vi "Load Ini FIle.vi"(8 "error in (no error)":errorcluster, 10 "Variant":variant, 11 "configuration file path":path) -> (0 "error out":errorcluster, 3 "Array":string[](array[string]))   [LabVIEW 2019, in "Configuration.lvlib"]
doc: "This method decodes a ini file based on an example typedef."
uses:
  Configuration.lvlib
  <vilib>/Utility/config.llb/Read Key (U32).vi
  <vilib>/Utility/config.llb/Read Key (Boolean).vi
  <vilib>/Utility/config.llb/Read Key (String).vi
  <vilib>/Utility/config.llb/Read Key (Path).vi
  <vilib>/Utility/config.llb/Read Key (I32).vi
  <vilib>/Utility/config.llb/Read Key (Double).vi
  <vilib>/Utility/config.llb/NI_LVConfig.lvlib
  <vilib>/Utility/Data Type/NI_Data Type.lvlib
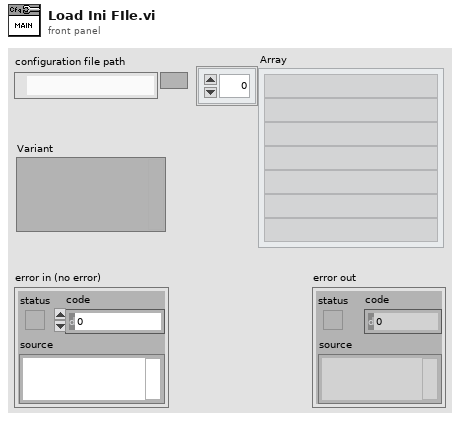
[diagram p1: front panel]
types:
  T1 = typedef "NI_LVConfig.lvlib/Config Data RefNum.ctl" = refnum<k1>
  T2 = typedef "NI_Data Type.lvlib/Data Type.ctl" = enum8{"Invalid Type", "Void", "I8", "I16", "I32", "I64", "U8", "U16", "U32", "U64", "Single Float", "Double Float", "Extended Float", "Single Complex", "Double Complex", "Extended Complex", "Enum U8", "Enum U16", "Enum U32", "Enum U64", "Single Float With Unit", "Double Float With Unit", "Extended Float With Unit", "Single Complex with Unit", "Double Complex with Unit", "Extended Complex with Unit", "Boolean", "String", "Path", "Picture", "Tag", "Array", "Cluster", "Variant", "LV Variant", "Waveform", "Timestamp", "Digital Waveform", "Digital Data", "ExpressData", "Refnum", "External Data", "VI", "Poly VI", "LabVIEW Class Instance", "Fixed Point", "Set Collection", "Map Collection"}
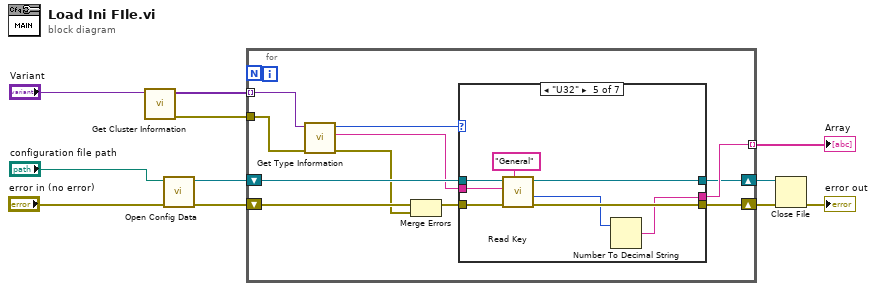
[diagram p0: block diagram]
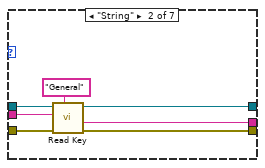
[diagram p3: hidden frame]
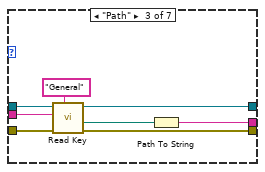
[diagram p4: hidden frame]
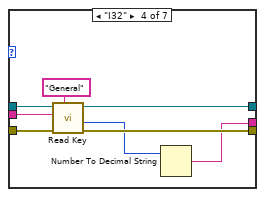
[diagram p5: hidden frame]
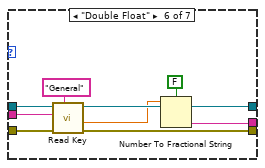
[diagram p6: hidden frame]
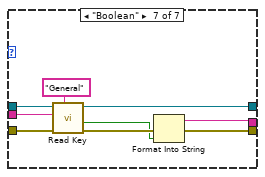
[diagram p7: hidden frame]
diagram:
  n1 = call <vilib>:"Get Cluster Information.vi"("variant"="Variant") -> ("error out"=w2:errorcluster, "cluster elements"=w3:variant[])  [unwired: 9 in]
  n2 = call <vilib>:"Open Config Data.vi"("error in (no error)"="error in (no error)", "configuration file path"="configuration file path") -> ("error out"=w10:errorcluster, "refnum"=w11:T1)  [unwired: 7 in, 1 out]
  n3 = for {
    shift-right: [w20] -> w8
    shift-left: w10 -> [w21]
    tunnel: [w19] -> w6 mode=indexing
    shift-right: [w18] -> w4
    shift-left: w11 -> [w22]
    tunnel: w3 -> [w14] mode=indexing
    tunnel: w2 -> [w15]
    n4 = call <vilib>:"Get Type Information.vi"("error in (no error)"=w15, "variant"=w14) -> ("error out"=w12:errorcluster, "name"=w16:string, "type"=w17:T2)  [unwired: 5 in, 2 out]
    n5 = Merge Errors(w21, w12) -> (w13:errorcluster)
    n6 = case shown="\"U32\"" w17 {
      tunnel: w22 -> [w23 w31 w39 w47 w55 w64 w73]
      tunnel: w13 -> [w24 w30 w38 w46 w54 w63 w72]
      tunnel: [w24 w28 w36 w44 w52 w61 w68] -> w20
      tunnel: w16 -> [_ w27 w35 w43 w51 w60 w69]
      tunnel: [_ w26 w32 w41 w49 w58 w66] -> w19
      tunnel: [w23 w25 w33 w42 w50 w59 w65] -> w18
      frame Default {
      }
      frame "String" {
        n7 = call-poly <vilib>:"Read Key.vi"("section"="General", "error in (no error)"=w30, "key"=w27, "refnum"=w31) -> ("error out"=w28:errorcluster, "value"=w26:string, "refnum out"=w25:T1)  [unwired: 4 in, 1 out]
      }
      frame "Path" {
        n8 = call-poly <vilib>:"Read Key.vi"("section"="General", "error in (no error)"=w38, "key"=w35, "refnum"=w39) -> ("error out"=w36:errorcluster, "value"=w34:path, "refnum out"=w33:T1)  [unwired: 4 in, 1 out]
        n9 = Path To String(path=w34) -> (string=w32:string)
      }
      frame "I32" {
        n10 = call-poly <vilib>:"Read Key.vi"("section"="General", "error in (no error)"=w46, "key"=w43, "refnum"=w47) -> ("error out"=w44:errorcluster, "value"=w40:i32, "refnum out"=w42:T1)  [unwired: 4 in, 1 out]
        n11 = Number To Decimal String(number=w40) -> (decimal integer string=w41:string)  [unwired: 1 in]
      }
      frame "U32" {
        n12 = call-poly <vilib>:"Read Key.vi"("section"="General", "error in (no error)"=w54, "key"=w51, "refnum"=w55) -> ("error out"=w52:errorcluster, "value"=w48:u32, "refnum out"=w50:T1)  [unwired: 4 in, 1 out]
        n13 = Number To Decimal String(number=w48) -> (decimal integer string=w49:string)  [unwired: 1 in]
      }
      frame "Double Float" {
        n14 = call-poly <vilib>:"Read Key.vi"("section"="General", "error in (no error)"=w63, "key"=w60, "refnum"=w64) -> ("error out"=w61:errorcluster, "value"=w56:dbl, "refnum out"=w59:T1)  [unwired: 4 in, 1 out]
        n15 = Number To Fractional String(use system decimal point (T)=FALSE, number=w56) -> (F-format string=w58:string)  [unwired: 2 in]
      }
      frame "Boolean" {
        n16 = call-poly <vilib>:"Read Key.vi"("section"="General", "error in (no error)"=w72, "key"=w69, "refnum"=w73) -> ("error out"=w70:errorcluster, "value"=w67:bool, "refnum out"=w65:T1)  [unwired: 4 in, 1 out]
        n17 = Format Into String(error in=w70, w67) -> (resulting string=w66:string, error out=w68:errorcluster)  [unwired: 2 in]
      }
    }
  }
  "Array" <- w6
  n18 = Close File(refnum=w4, error in=w8) -> (error out=→"error out":errorcluster)  [unwired: 1 out]
